vi "Plot Generation vs Fitness.vi"(8 "error in (no error)":errorcluster, 10 "OSSP_Problem.lvclass":refnum<class "OSSP_Problem.lvclass">, 11 "GA in":refnum<class "GA.lvclass">) -> (0 "error out":errorcluster, 2 "Picture":picture, 3 "GA out":refnum<class "GA.lvclass">)   [LabVIEW 2013, in "GA.lvclass"]
uses:
  GA.lvclass
  OSSP_Problem.lvclass
  GA.lvclass/GA.ctl
  <vilib>/Heliosphere Research LLC/Advanced Plotting Toolkit/api_plotting/LineProperties.ctl
  <vilib>/Heliosphere Research LLC/Advanced Plotting Toolkit/properties/Line.ctl
  <vilib>/Heliosphere Research LLC/Advanced Plotting Toolkit/properties/Line_Style.ctl
  <vilib>/Heliosphere Research LLC/Advanced Plotting Toolkit/typedefs/PlotColor.ctl
  <vilib>/Heliosphere Research LLC/Advanced Plotting Toolkit/properties/Marker.ctl
  <vilib>/Heliosphere Research LLC/Advanced Plotting Toolkit/properties/Marker_Style.ctl
  <vilib>/Heliosphere Research LLC/Advanced Plotting Toolkit/properties/Display.ctl
  <vilib>/Heliosphere Research LLC/Advanced Plotting Toolkit/api_figure/TicksProperties.ctl
  <vilib>/Heliosphere Research LLC/Advanced Plotting Toolkit/properties/Text.ctl
  <vilib>/Heliosphere Research LLC/Advanced Plotting Toolkit/properties/Text_FontSize.ctl
  <vilib>/Heliosphere Research LLC/Advanced Plotting Toolkit/properties/Text_FontStyle.ctl
  <vilib>/Heliosphere Research LLC/Advanced Plotting Toolkit/api_annotations/ShapeProperties.ctl
  GA_Operation_To_MachineJobTuple.vi
  Find Gaps On Particular Machine.vi
  GA_Check_Other_Machines.vi
  GA_Schedule_Job.vi
  GA_Find_Job_On_Other_Machines.vi
  GA_Increment_NumberofJobsOn Machine_ByOne.vi
  <vilib>/Heliosphere Research LLC/Advanced Plotting Toolkit/Advanced Plotting Toolkit.lvlib
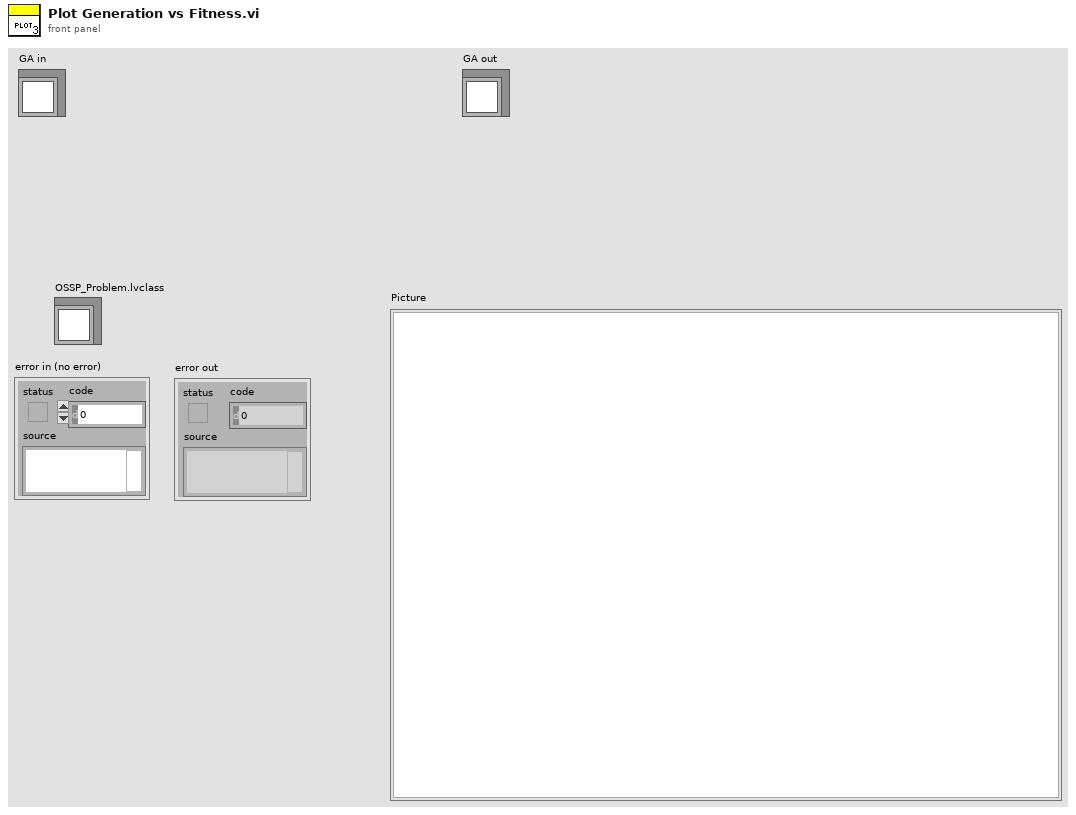
[diagram p1: front panel]
types:
  T1 = typedef "Advanced Plotting Toolkit.lvlib/LineProperties.ctl" = cluster{"Line":T2, "Marker":T5, "Display":T7}
  T2 = typedef "Advanced Plotting Toolkit.lvlib/Line.ctl" = cluster{"Style":T3, "Color":T4, "Width":sgl}
  T3 = typedef "Advanced Plotting Toolkit.lvlib/Line_Style.ctl" = enum16{"Automatic", "Solid", "Dashed", "Dotted", "Dash-dot", "Invisible"}
  T4 = typedef "Advanced Plotting Toolkit.lvlib/PlotColor.ctl" = u32
  T5 = typedef "Advanced Plotting Toolkit.lvlib/Marker.ctl" = cluster{"Style":T6, "Color":T4, "Size":dbl}
  T6 = typedef "Advanced Plotting Toolkit.lvlib/Marker_Style.ctl" = enum16{"Automatic", "Circle", "Square", "Triangle", "Diamond", "Star", "Invisible"}
  T7 = typedef "Advanced Plotting Toolkit.lvlib/Display.ctl" = cluster{"Alpha":dbl, "Z Order":dbl}
  T8 = typedef "Advanced Plotting Toolkit.lvlib/TicksProperties.ctl" = cluster{"Text":T9}
  T9 = typedef "Advanced Plotting Toolkit.lvlib/Text.ctl" = cluster{"Color":T4, "Background Color":T4, "Font Size (points)":T10, "Font Style":T11, "Rotation Angle":dbl}
  T10 = typedef "Advanced Plotting Toolkit.lvlib/Text_FontSize.ctl" = i32
  T11 = typedef "Advanced Plotting Toolkit.lvlib/Text_FontStyle.ctl" = enum16{"Automatic", "Normal", "Italic", "Bold"}
  T12 = typedef "Advanced Plotting Toolkit.lvlib/ShapeProperties.ctl" = cluster{"Color":T4, "Line":T2, "Display":T7}
  T13 = typedef "Population Statistics.ctl" = cluster{"Min":u16, "Max":u16, "Mean":dbl}
  T14 = typedef "Plot Type.ctl" = enum16{"No Plot", "Min Max Mean Plot", "Gannt Chart"}
  T15 = typedef "Solution.ctl" = cluster{"Schedule":u16[], "Fitness":u16, "Fitness Valid?":bool}
  T16 = typedef "Advanced Plotting Toolkit.lvlib/PlotID.ctl" = i32
  T17 = typedef "GanntChart_Element.ctl" = cluster{"Operation Number":i32, "Job Number":i32, "Start Time":i32, "Procesing Time":u16, "End Time":i32}
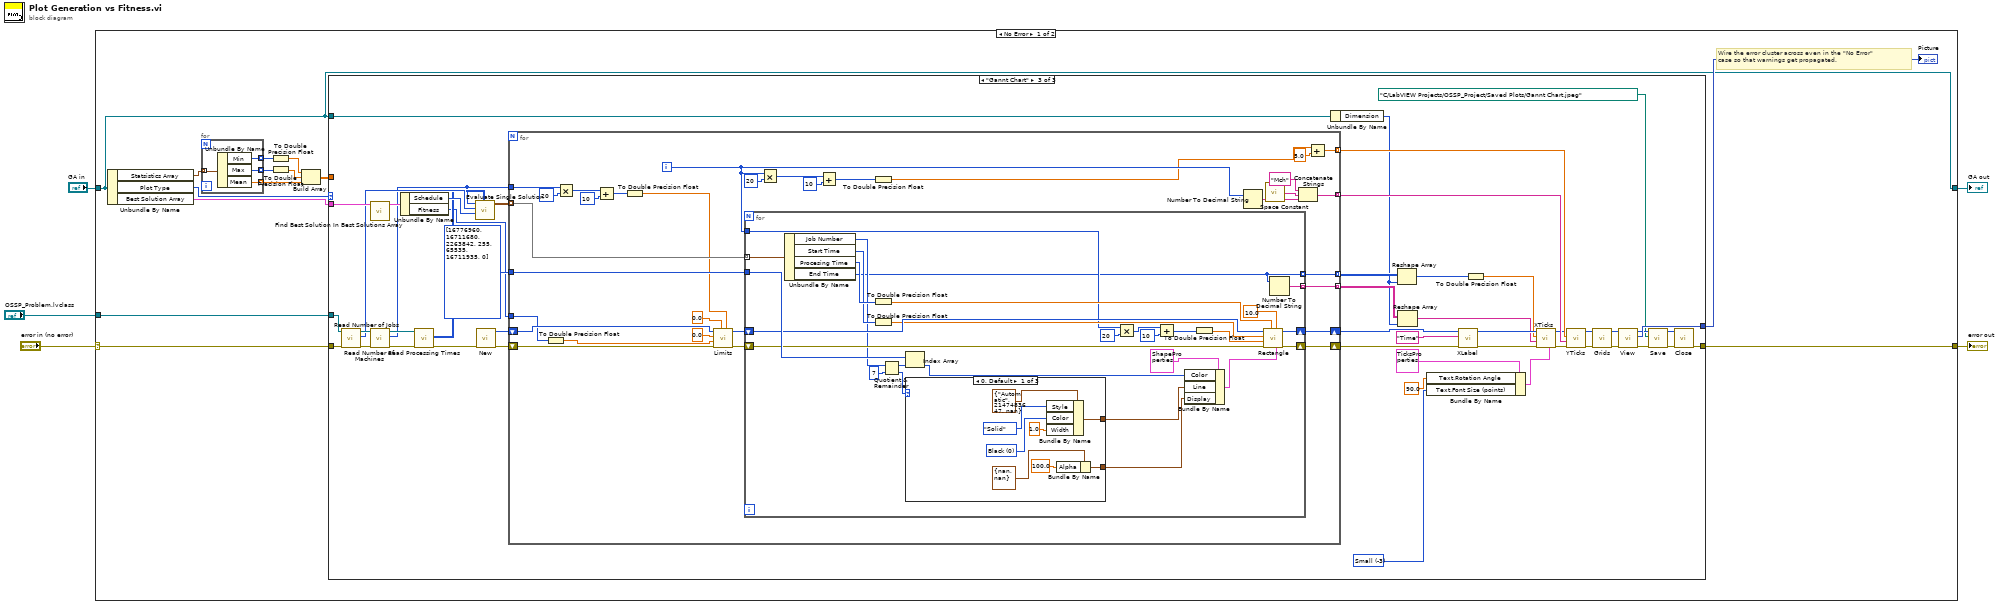
[diagram p0: block diagram]
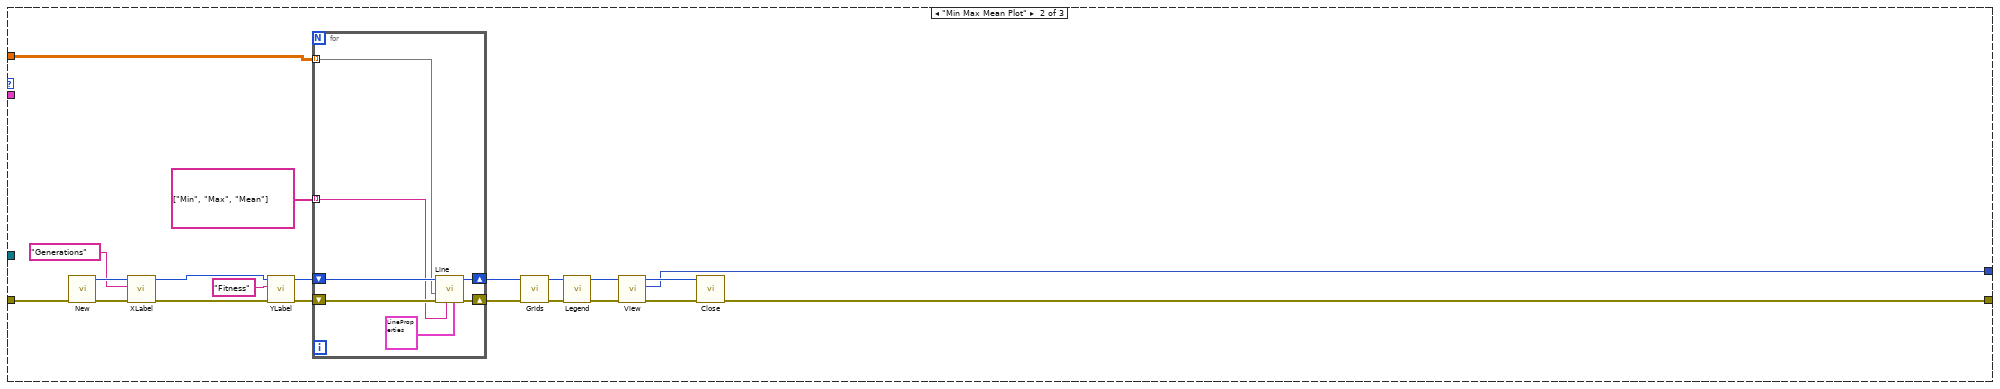
[diagram p3: hidden frame]
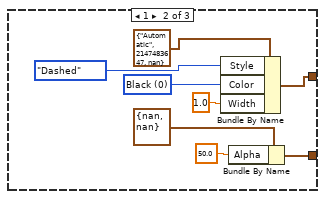
[diagram p4: hidden frame]
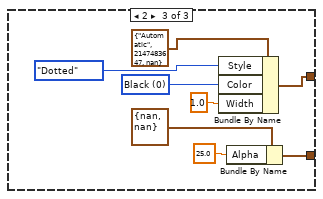
[diagram p5: hidden frame]
diagram:
  n1 = case shown="No Error" "error in (no error)" {
    selector: "error in (no error)" -> [w10 w187]
    tunnel: [w18 w187] -> w4
    tunnel: [w6 w186] -> w2
    tunnel: "GA in" -> [w6 w186]
    tunnel: "OSSP_Problem.lvclass" -> [w7 _]
    frame No Error {
      # "Wire the error cluster across even in the \"No Error\"\ncase so that warnings get propagated."
      n2 = Unbundle By Name(w6) -> ("Statsistics Array"=w17:T13[], "Plot Type"=w9:T14, "Best Solution Array"=w8:T15[])
      n3 = for {
        tunnel: [w182] -> w16 mode=indexing
        tunnel: w17 -> [w185] mode=indexing
        tunnel: [w184] -> w15 mode=indexing
        tunnel: [w183] -> w12 mode=indexing
        n4 = Unbundle By Name(w185) -> ("Min"=w182:u16, "Max"=w184:u16, "Mean"=w183:dbl)
      }
      n5 = To Double Precision Float(number=w16) -> (double precision float=w14:dbl[])
      n6 = To Double Precision Float(number=w15) -> (double precision float=w13:dbl[])
      n7 = Build Array(w14, w13, w12) -> (w11:dbl[][])
      n8 = case shown="\"Gannt Chart\"" w9 {
        tunnel: [_ w39 w94] -> w19
        tunnel: [w20 w38 w95] -> w18
        tunnel: w11 -> [_ w37 _]
        tunnel: w10 -> [w20 w21 w90]
        tunnel: w8 -> [_ _ w93]
        tunnel: w7 -> [_ _ w86]
        tunnel: w6 -> [_ _ w67]
        frame "No Plot", Default {
        }
        frame "Min Max Mean Plot" {
          n9 = call <vilib>:"New.vi"("error in (no error)"=w21) -> ("error out"=w34:errorcluster, "Plot ID"=w35:T16)  [unwired: 9 in]
          n10 = call <vilib>:"XLabel.vi"("error in (no error)"=w34, "Label"="Generations", "Plot ID"=w35) -> ("error out"=w30:errorcluster, "Plot ID out"=w32:T16)  [unwired: 7 in]
          n11 = call <vilib>:"YLabel.vi"("error in (no error)"=w30, "Label"="Fitness", "Plot ID"=w32) -> ("error out"=w28:errorcluster, "Plot ID out"=w29:T16)  [unwired: 7 in]
          n12 = for {
            tunnel: w37 -> [w44] mode=indexing
            shift-right: [w46] -> w27
            shift-left: w29 -> [w47]
            shift-right: [w45] -> w26
            shift-left: w28 -> [w48]
            tunnel: string[] ["Min", "Max", "Mean"] -> [w43] mode=indexing
            n13 = call <vilib>:"Line.vi"("Properties"=T1 {"Line"={"Style"=enum."Automatic", "Color"=2147483647, "Width"=nan}, "Marker"={"Style"=enum."Automatic", "Color"=2147483647, "Size"=nan}, "Display"={"Alpha"=nan, "Z Order"=nan}}, "Legend Title"=w43, "error in (no error)"=w48, "Y Data"=w44, "Plot ID"=w47) -> ("error out"=w45:errorcluster, "Plot ID out"=w46:T16)  [unwired: 5 in]
          }
          n14 = call <vilib>:"Grids.vi"("error in (no error)"=w26, "Plot ID"=w27) -> ("error out"=w23:errorcluster, "Plot ID Out"=w25:T16)  [unwired: 8 in]
          n15 = call <vilib>:"Legend.vi"("error in (no error)"=w23, "Plot ID"=w25) -> ("error out"=w22:errorcluster, "Plot ID Out"=w24:T16)  [unwired: 8 in]
          n16 = call <vilib>:"View.vi"("error in (no error)"=w22, "Plot ID"=w24) -> ("error out"=w40:errorcluster, "Picture"=w39:picture, "Plot ID Out"=w41:T16)  [unwired: 7 in]
          n17 = call <vilib>:"Close.vi"("error in (no error)"=w40, "Plot ID"=w41) -> ("error out"=w38:errorcluster)  [unwired: 9 in]
        }
        frame "Gannt Chart" {
          w49 = T10 -3 items=["Automatic"=0, "XX-Small"=-1, "X-Small"=-2, "Small"=-3, "Medium"=-4, "Large"=-5, "X-Large"=-6, "XX-Large"=-7] ("Text.Font Size (points)")
          w80 = T4[] [16776960, 16711680, 2263842, 255, 65535, 16711935, 0] items=["Automatic"=2147483647, "Black"=0, "White"=16777215, "Red"=16711680, "Green"=2263842, "Blue"=255, "Cyan"=65535, "Magenta"=16711935, "Yellow"=16776960]
          n18 = call-dynamic "Read Number of Jobs.vi"("error in (no error)"=w90, "OSSP_Problem in"=w86) -> ("error out"=w89:errorcluster, "Number of Jobs"=w83:i32, "OSSP_Problem out"=w85:refnum<class "OSSP_Problem.lvclass">)  [unwired: 7 in]
          n19 = call "Find Best Solution In Best Solutions Array.vi"("Best Solution Array"=w93) -> ("Best Solution"=w92:T15)  [unwired: 10 in]
          n20 = call-dynamic "Read Number of Machines.vi"("error in (no error)"=w89, "OSSP_Problem in"=w85) -> ("error out"=w88:errorcluster, "Number of Machines"=w79:i32, "OSSP_Problem out"=w84:refnum<class "OSSP_Problem.lvclass">)  [unwired: 7 in]
          n21 = Unbundle By Name(w92) -> ("Schedule"=w91:u16[], "Fitness"=w78:u16)
          n22 = call-dynamic "Read Processing Times.vi"("error in (no error)"=w88, "OSSP_Problem in"=w84) -> ("error out"=w87:errorcluster, "Processing Times"=w82:u16[][])  [unwired: 7 in, 1 out]
          n23 = call "Evaluate Single Solution.vi"("Processing Times (Rows Mach.Cols Jobs)"=w82, "Schedule"=w91, "Number of Jobs"=w83, "Number of Machines"=w79) -> ("Gannt Chart Out"=w81:T17[][])  [unwired: 7 in]
          n24 = call <vilib>:"New.vi"("error in (no error)"=w87) -> ("error out"=w96:errorcluster, "Plot ID"=w97:T16)  [unwired: 9 in]
          n25 = for {
            shift-right: [w129] -> w76
            shift-left: w96 -> [w125]
            shift-right: [w128] -> w77
            shift-left: w97 -> [w123]
            tunnel: w81 -> [w127] mode=indexing
            tunnel: w80 -> [w126]
            tunnel: w79 -> [w122]
            tunnel: w78 -> [w121]
            tunnel: [w110] -> w70 mode=indexing
            tunnel: [w100] -> w69 mode=indexing
            tunnel: [w99] -> w68 mode=indexing
            tunnel: [w98] -> w62 mode=indexing
            i -> [w103]
            n26 = To Double Precision Float(number=w121) -> (double precision float=w113:dbl)
            n27 = Multiply(x=w122, y=20) -> (x*y=w119:i32)
            n28 = Add(x=w119, y=10) -> (x+y=w117:i32)
            n29 = To Double Precision Float(number=w117) -> (double precision float=w108:dbl)
            n30 = call <vilib>:"Limits.vi"("Y Max"=w108, "Y Min"=0.0, "error in (no error)"=w125, "X Max"=w113, "X Min"=0.0, "Plot ID"=w123) -> ("error out"=w124:errorcluster, "Plot ID Out"=w115:T16)  [unwired: 4 in]
            n31 = for {
              shift-right: [w157] -> w129
              shift-left: w124 -> [w153]
              shift-right: [w156] -> w128
              shift-left: w115 -> [w152]
              tunnel: w127 -> [w155] mode=indexing
              tunnel: w126 -> [w154]
              tunnel: w103 -> [w138]
              tunnel: [w131] -> w99 mode=indexing
              tunnel: [w130] -> w98 mode=indexing
              n32 = Unbundle By Name(w155) -> ("Job Number"=w136:i32, "Start Time"=w145:i32, "Procesing Time"=w147:u16, "End Time"=w131:i32)
              n33 = To Double Precision Float(number=w147) -> (double precision float=w146:dbl)
              n34 = To Double Precision Float(number=w145) -> (double precision float=w144:dbl)
              n35 = Quotient & Remainder(x=w136, y=7) -> (x-y*floor(x/y)=w134:i32, floor(x/y)=w133:i32)
              n36 = Index Array(array=w154, index=w134) -> (element=w149:T4)
              n37 = case shown="0, Default" w133 {
                tunnel: [w161 w169 w177] -> w137
                tunnel: [w158 w166 w174] -> w132
                frame 0, Default {
                  w163 = T4 0 items=["Automatic"=2147483647, "Black"=0, "White"=16777215, "Red"=16711680, "Green"=2263842, "Blue"=255, "Cyan"=65535, "Magenta"=16711935, "Yellow"=16776960] ("Color")
                  n38 = Bundle By Name(cluster=T2 {"Style"=enum."Automatic", "Color"=2147483647, "Width"=nan} ("Line"), "Style"=Line_Style."Solid", "Color"=w163, "Width"=sgl 1.0) -> (w161:T2)
                  n39 = Bundle By Name(cluster=T7 {"Alpha"=nan, "Z Order"=nan} ("Display"), "Alpha"=100.0) -> (w158:T7)
                }
                frame 1 {
                  w171 = T4 0 items=["Automatic"=2147483647, "Black"=0, "White"=16777215, "Red"=16711680, "Green"=2263842, "Blue"=255, "Cyan"=65535, "Magenta"=16711935, "Yellow"=16776960] ("Color")
                  n40 = Bundle By Name(cluster=T2 {"Style"=enum."Automatic", "Color"=2147483647, "Width"=nan} ("Line"), "Style"=Line_Style."Dashed", "Color"=w171, "Width"=sgl 1.0) -> (w169:T2)
                  n41 = Bundle By Name(cluster=T7 {"Alpha"=nan, "Z Order"=nan} ("Display"), "Alpha"=50.0) -> (w166:T7)
                }
                frame 2 {
                  w179 = T4 0 items=["Automatic"=2147483647, "Black"=0, "White"=16777215, "Red"=16711680, "Green"=2263842, "Blue"=255, "Cyan"=65535, "Magenta"=16711935, "Yellow"=16776960] ("Color")
                  n42 = Bundle By Name(cluster=T2 {"Style"=enum."Automatic", "Color"=2147483647, "Width"=nan} ("Line"), "Style"=Line_Style."Dotted", "Color"=w179, "Width"=sgl 1.0) -> (w177:T2)
                  n43 = Bundle By Name(cluster=T7 {"Alpha"=nan, "Z Order"=nan} ("Display"), "Alpha"=25.0) -> (w174:T7)
                }
              }
              n44 = Multiply(x=w138, y=20) -> (x*y=w142:i32)
              n45 = Add(x=w142, y=10) -> (x+y=w140:i32)
              n46 = Bundle By Name(cluster=T12 {"Color"=2147483647, "Line"={"Style"=enum."Automatic", "Color"=2147483647, "Width"=nan}, "Display"={"Alpha"=nan, "Z Order"=nan}} ("Properties"), "Color"=w149, "Line"=w137, "Display"=w132) -> (w150:T12)
              n47 = To Double Precision Float(number=w140) -> (double precision float=w139:dbl)
              n48 = call <vilib>:"Rectangle.vi"("Properties"=w150, "Height"=10.0, "Width"=w146, "error in (no error)"=w153, "Y Position"=w139, "X Position"=w144, "Plot ID"=w152) -> ("error out"=w157:errorcluster, "Plot ID Out"=w156:T16)  [unwired: 3 in]
              n49 = Number To Decimal String(number=w131) -> (decimal integer string=w130:string)  [unwired: 1 in]
            }
            n50 = Multiply(x=w103, y=20) -> (x*y=w106:i32)
            n51 = Add(x=w106, y=10) -> (x+y=w104:i32)
            n52 = To Double Precision Float(number=w104) -> (double precision float=w102:dbl)
            n53 = Number To Decimal String(number=w103) -> (decimal integer string=w109:string)  [unwired: 1 in]
            n54 = call <vilib>:"Space Constant.vi"() -> ("String"=w111:string)
            n55 = Concatenate Strings("Mch", w111, w109) -> (w110:string)
            n56 = Add(x=w102, y=5.0) -> (x+y=w100:dbl)
          }
          n57 = Unbundle By Name(w67) -> ("Dimension"=w61:i32)
          n58 = Reshape Array(w68, w61) -> (w59:i32[])
          n59 = Reshape Array(w62, w61) -> (w60:string[])
          n60 = Bundle By Name(cluster=T8 {"Text"={"Color"=2147483647, "Background Color"=2147483647, "Font Size (points)"=0, "Font Style"=enum."Automatic", "Rotation Angle"=nan}} ("Properties"), "Text.Rotation Angle"=90.0, "Text.Font Size (points)"=w49) -> (w55:T8)
          n61 = call <vilib>:"XLabel.vi"("error in (no error)"=w76, "Label"="Time", "Plot ID"=w77) -> ("error out"=w64:errorcluster, "Plot ID out"=w66:T16)  [unwired: 7 in]
          n62 = To Double Precision Float(number=w59) -> (double precision float=w58:dbl[])
          n63 = call <vilib>:"XTicks.vi"("Properties"=w55, "error in (no error)"=w64, "Tick Labels"=w60, "Tick Locations"=w58, "Plot ID"=w66) -> ("error out"=w63:errorcluster, "Plot ID Out"=w65:T16)  [unwired: 5 in]
          n64 = call <vilib>:"YTicks.vi"("error in (no error)"=w63, "Tick Labels"=w70, "Tick Locations"=w69, "Plot ID"=w65) -> ("error out"=w72:errorcluster, "Plot ID Out"=w71:T16)  [unwired: 6 in]
          n65 = call <vilib>:"Grids.vi"("error in (no error)"=w72, "Plot ID"=w71) -> ("error out"=w75:errorcluster, "Plot ID Out"=w73:T16)  [unwired: 8 in]
          n66 = call <vilib>:"View.vi"("error in (no error)"=w75, "Plot ID"=w73) -> ("error out"=w54:errorcluster, "Picture"=w94:picture, "Plot ID Out"=w52:T16)  [unwired: 7 in]
          n67 = call <vilib>:"Save.vi"("error in (no error)"=w54, "Path"=path "C:/LabVIEW Projects/OSSP_Project/Saved Plots/Gannt Chart.jpeg", "Plot ID In"=w52) -> ("error out"=w53:errorcluster, "Plot ID Out"=w51:T16)  [unwired: 7 in]
          n68 = call <vilib>:"Close.vi"("error in (no error)"=w53, "Plot ID"=w51) -> ("error out"=w95:errorcluster)  [unwired: 9 in]
        }
      }
      "Picture" <- w19
    }
    frame Error {
    }
  }
  "error out" <- w4
  "GA out" <- w2
